vi "AI & AO Synchronization.vi"() -> ()   [LabVIEW 2009, in "MicroDAQ.lvlib"]
uses:
  <instrlib>/MicroDAQ/MicroDAQ.lvlib
  <instrlib>/MicroDAQ/Tools/Analog mode.ctl
  <instrlib>/MicroDAQ/Tools/Analo Range Enum.ctl
  <instrlib>/MicroDAQ/Tools/Analog Channel Enum.ctl
  <instrlib>/MicroDAQ/Tools/Analog input type enum.ctl
  <instrlib>/MicroDAQ/Tools/Analog input Channel enum.ctl
  <instrlib>/MicroDAQ/Tools/External start trigger source.ctl
  <instrlib>/MicroDAQ/Channel/Analog Input/Read NChan NSamp 2D SGL.vi
  <instrlib>/MicroDAQ/Channel/Analog Input/Triggering External start.vi
  <instrlib>/MicroDAQ/Channel/Analog Input/AI Configure Channel.vi
  <instrlib>/MicroDAQ/Channel/Analog Output/Write NChan NSamp 1D Waveform.vi
  <instrlib>/MicroDAQ/Channel/Analog Output/AO Configure Channel.vi
  <instrlib>/MicroDAQ/Channel/Analog Input/Analog Input.lvclass
  <instrlib>/MicroDAQ/Channel/Analog Output/Analog output.lvclass
  <vilib>/measure/NI_MABase.lvlib
panel:
  in  "Sampe Rate":dbl=1000.0
  in  "Samples per channel":dbl=1.0
  out "AI read finish":u32
  out "AI read ready start":u32
  out "AO generation start":u32
  out "AO wait start":u32
  in  "IP address":string="10.10.1.1"
  out "Waveform Graph 2":waveform(dbl)[](graph)=[{"t0"=timestamp(0 s since 1904-01-01), "dt"=0.001, "Y"=[]}]
  out "Waveform Graph":dbl[][](graph)
  # "Device settings"
  # "* All input and output channels settings have been preconfigured as \nconstans to symplify example."
  # "this time should trigger AI start,\nand AI should measure 1000 ms\nand return. So in theory \nAI read finish = AO generation start + 1000ms"
  # "Output signal"
  # "Input signal"
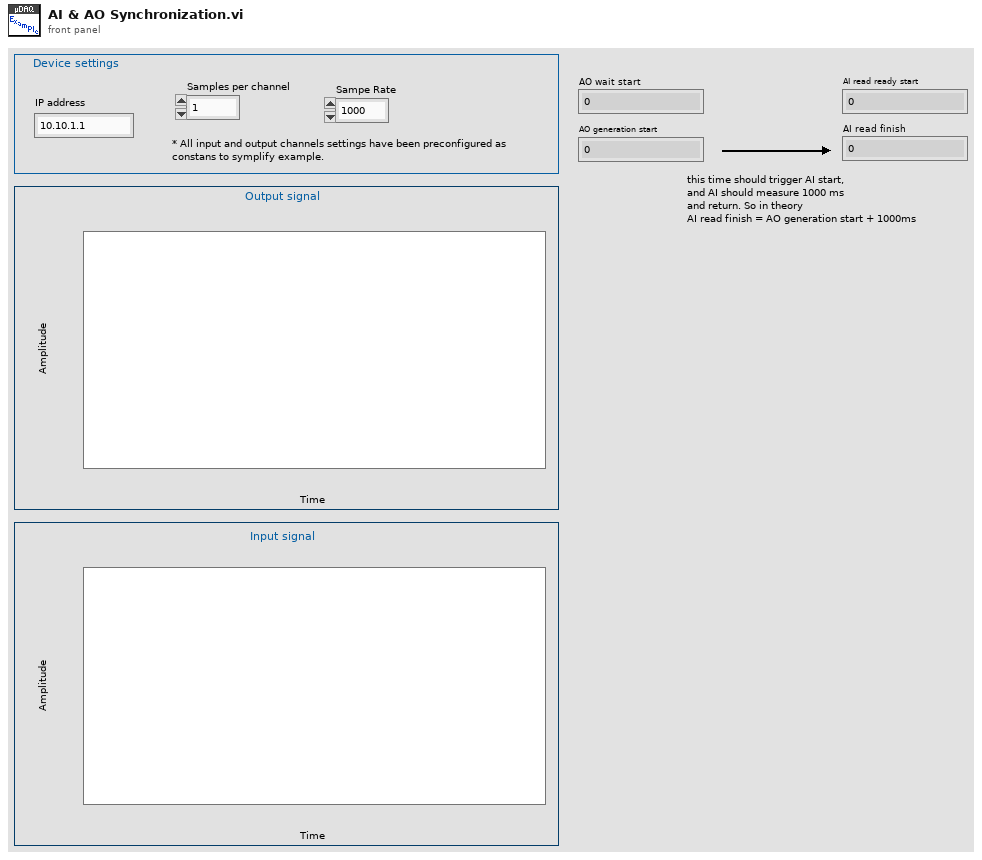
[diagram p1: front panel]
types:
  T1 = typedef "MicroDAQ.lvlib/External start trigger source.ctl" = u16
  T2 = cluster{"Waveform Type":enum16{"Sine Wave", "Triangle Wave", "Square Wave", "Sawtooth Wave"}, "Amplitude":dbl, "Frequency":dbl}[]
  T3 = typedef "MicroDAQ.lvlib/Analog input Channel enum.ctl" = enum16{"None", "AI1", "AI2", "AI3", "AI4", "AI5", "AI6", "AI7", "AI8", "AI9", "AI10", "AI11", "AI12", "AI13", "AI14", "AI15", "AI16"}
  T4 = typedef "MicroDAQ.lvlib/Analo Range Enum.ctl" = enum16{"±10V", "0-10V", "±5V", "0-5V", "±5.12V", "±2.56V", "±2.5V", "±2V", "±1.24V", "±0.64V"}
  T5 = typedef "MicroDAQ.lvlib/Analog input type enum.ctl" = enum16{"Single-ended", "Differential"}
  T6 = typedef "MicroDAQ.lvlib/Analog Channel Enum.ctl" = enum16{"None", "AO1", "AO2", "AO3", "AO4", "AO5", "AO6", "AO7", "AO8", "AO9", "AO10", "AO11", "AO12", "AO13", "AO14", "AO15", "AO16"}
  T7 = typedef "MicroDAQ.lvlib/Analog mode.ctl" = enum16{"Periodic", "Stream"}
  T8 = enum16{"Sine Wave", "Triangle Wave", "Square Wave", "Sawtooth Wave"}
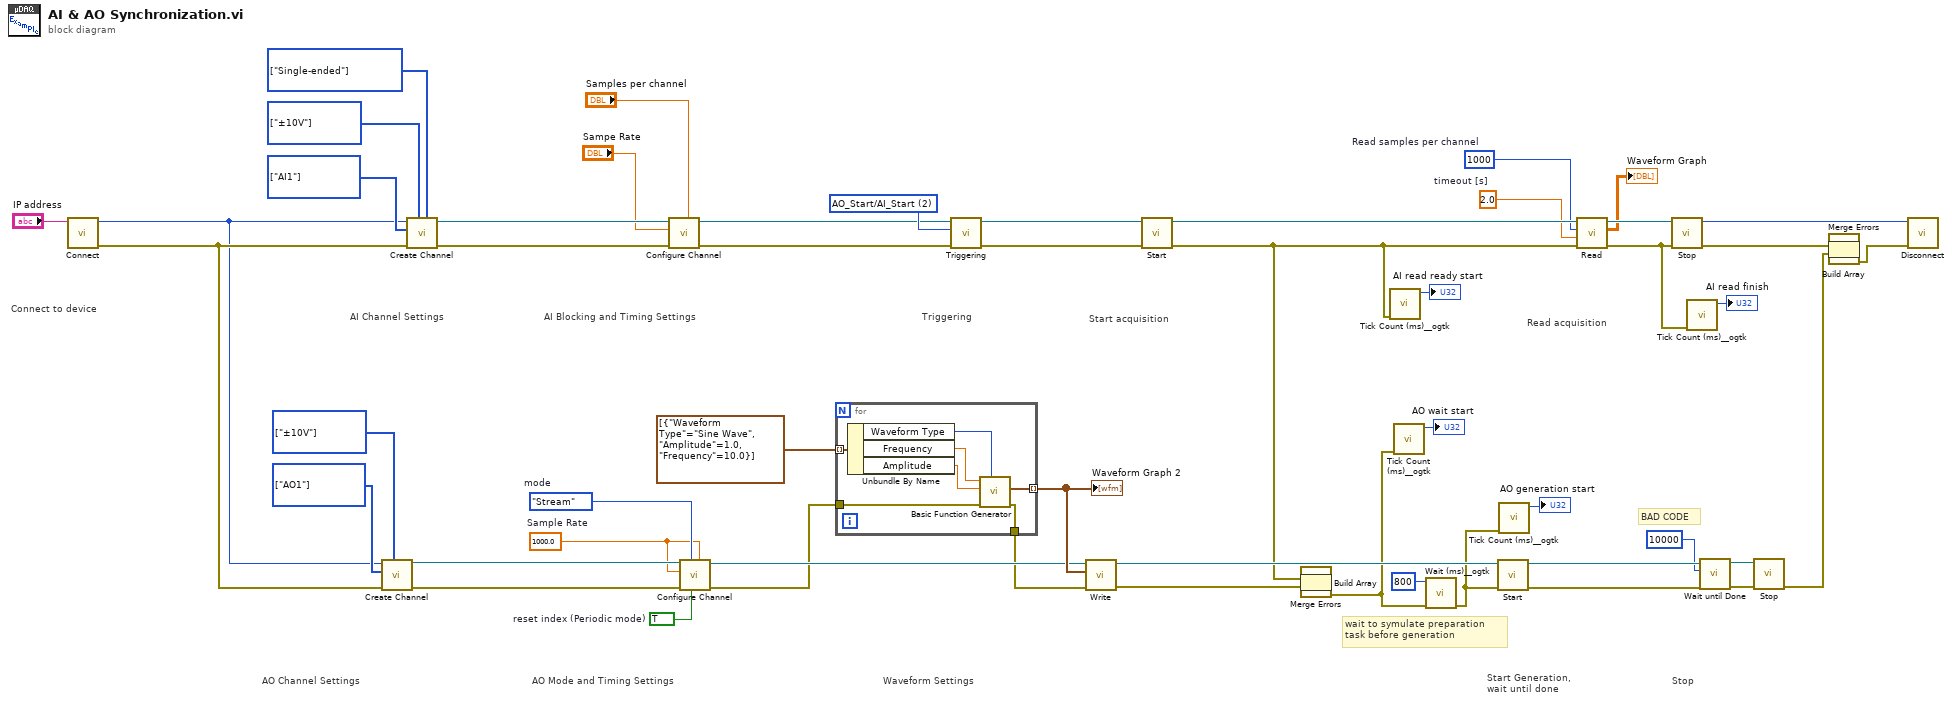
[diagram p0: block diagram]
diagram:
  w20 = T1 2 items=["AO_Start/AI_Start"=2, "DSP_Start"=3] ("source")
  w21 = 2.0  # timeout [s]
  w47 = 1000  # Read samples per channel
  w49 = T3[] [enum."AI1"] items=["None", "AI1", "AI2", "AI3", "AI4", "AI5", "AI6", "AI7", "AI8", "AI9", "AI10", "AI11", "AI12", "AI13", "AI14", "AI15", "AI16"] ("Physical channels")
  w48 = T4[] [enum."±10V"] items=["±10V", "0-10V", "±5V", "0-5V", "±5.12V", "±2.56V", "±2.5V", "±2V", "±1.24V", "±0.64V"] ("Ranges")
  w50 = T5[] [enum."Single-ended"] items=["Single-ended", "Differential"] ("Input terminals configurations")
  w7 = 1000.0  # Sample Rate
  w43 = T6[] [enum."AO1"] items=["None", "AO1", "AO2", "AO3", "AO4", "AO5", "AO6", "AO7", "AO8", "AO9", "AO10", "AO11", "AO12", "AO13", "AO14", "AO15", "AO16"] ("Physical channels 2")
  w42 = T4[] [enum."±10V"] items=["±10V", "0-10V", "±5V", "0-5V", "±5.12V", "±2.56V", "±2.5V", "±2V", "±1.24V", "±0.64V"] ("Ranges 2")
  w38 = TRUE  # reset index (Periodic mode)
  w39 = Analog_mode."Stream"  # mode
  # "wait to symulate preparation \ntask before generation"
  # "BAD CODE"
  # "Start Generation,\nwait until done"
  # "Stop"
  # "Waveform Settings"
  # "AO Mode and Timing Settings"
  # "AO Channel Settings"
  # "Triggering"
  # "Connect to device"
  # "Read acquisition"
  # "Start acquisition"
  # "AI Blocking and Timing Settings"
  # "AI Channel Settings"
  n1 = call <instrlib>:"Connect.vi"("IP address"="IP address") -> ("error out"=w32:errorcluster, "connection ID"=w31:i32)  [unwired: 9 in]
  n2 = call-poly <instrlib>:"Create Channel.vi"("Ranges"=w42, "error in (no error)"=w32, "Phisical channels"=w43, "Connection ID"=w31) -> ("error out"=w40:errorcluster, "Task Out"=w41:refnum<class "Analog output.lvclass">)  [unwired: 6 in]
  n3 = call-poly <instrlib>:"Create Channel.vi"("Input terminals configurations"=w50, "Ranges"=w48, "error in (no error)"=w32, "Phisical channels"=w49, "connection ID"=w31) -> ("error out"=w54:errorcluster, "Task Out"=w4:refnum<class "Analog Input.lvclass">)  [unwired: 5 in]
  n4 = call-poly <instrlib>:"Configure Channel.vi"("Samples per channel"="Samples per channel", "error in (no error)"=w54, "Sampe Rate"="Sampe Rate", "MicroDAQ.lvlib:Analog Input.lvclass"=w4) -> ("error out"=w22:errorcluster, "MicroDAQ.lvlib:Analog Input.lvclass out"=w3:refnum<class "Analog Input.lvclass">)  [unwired: 6 in]
  n5 = call-poly <instrlib>:"Configure Channel.vi"("Samples per channel"=w7, "Reset index (Periodic mode)"=w38, "Mode"=w39, "error in (no error)"=w40, "Sample rate"=w7, "Analog Output in"=w41) -> ("error out"=w29:errorcluster, "Analog Output out"=w30:refnum<class "Analog output.lvclass">)  [unwired: 4 in]
  n6 = for {
    tunnel: [w61] -> w19
    tunnel: T2 [{"Waveform Type"=enum."Sine Wave", "Amplitude"=1.0, "Frequency"=10.0}] ("Waveforms") -> [w60] mode=indexing
    tunnel: [w56] -> w36 mode=indexing
    tunnel: w29 -> [w55]
    n7 = Unbundle By Name(w60) -> ("Waveform Type"=w59:T8, "Frequency"=w58:dbl, "Amplitude"=w57:dbl)
    n8 = call <vilib>:"Basic Function Generator.vi"("signal type"=w59, "error in (no error)"=w55, "amplitude"=w57, "frequency"=w58) -> ("error out"=w61:errorcluster, "signal out"=w56:waveform(dbl))  [unwired: 5 in, 1 out]
  }
  "Waveform Graph 2" <- w36
  n9 = call-poly <instrlib>:"Triggering.vi"("error in (no error)"=w22, "source"=w20, "MicroDAQ.lvlib:Analog Input.lvclass"=w3) -> ("error out"=w44:errorcluster, "MicroDAQ.lvlib:Analog Input.lvclass out"=w45:refnum<class "Analog Input.lvclass">)  [unwired: 7 in]
  n10 = call-poly <instrlib>:"Write.vi"("error in (no error)"=w19, "data"=w36, "Analog Output in"=w30) -> ("error out"=w9:errorcluster, "Analog Output out"=w28:refnum<class "Analog output.lvclass">)  [unwired: 7 in]
  n11 = call-dynamic "Start.vi"("error in (no error)"=w44, "Analog Input in"=w45) -> ("error out"=w8:errorcluster, "Analog Input out"=w53:refnum<class "Analog Input.lvclass">)  [unwired: 8 in]
  n12 = Build Array(w8, w9) -> (w6:errorcluster[])
  n13 = call <vilib>:"Merge Errors.vi"("error array in"=w6) -> ("error out"=w16:errorcluster)  [unwired: 6 in]
  n14 = call <userlib>:"Tick Count (ms)__ogtk.vi"("error in (no error)"=w8) -> ("millisecond timer value"=→"AI read ready start":u32)  [unwired: 9 in, 1 out]
  n15 = call <userlib>:"Tick Count (ms)__ogtk.vi"("error in (no error)"=w16) -> ("millisecond timer value"=→"AO wait start":u32)  [unwired: 9 in, 1 out]
  n16 = call <userlib>:"Wait (ms)__ogtk.vi"("error in (no error)"=w16, "milliseconds to wait"=u32 800) -> ("error out"=w13:errorcluster)  [unwired: 8 in, 1 out]
  n17 = call-dynamic "Start.vi"("error in (no error)"=w13, "Analog Output in"=w28) -> ("error out"=w18:errorcluster, "Analog Output out"=w26:refnum<class "Analog output.lvclass">)  [unwired: 8 in]
  n18 = call <userlib>:"Tick Count (ms)__ogtk.vi"("error in (no error)"=w13) -> ("millisecond timer value"=→"AO generation start":u32)  [unwired: 9 in, 1 out]
  n19 = call-poly <instrlib>:"Read.vi"("error in (no error)"=w8, "timeout [s]"=w21, "number of samples per channel"=w47, "MicroDAQ.lvlib:Analog Input.lvclass"=w53) -> ("error out"=w10:errorcluster, "Values"=→"Waveform Graph":dbl[][], "MicroDAQ.lvlib:Analog Input.lvclass out"=w52:refnum<class "Analog Input.lvclass">)  [unwired: 4 in, 1 out]
  n20 = call-dynamic "Stop.vi"("error in (no error)"=w10, "Analog Input in"=w52) -> ("error out"=w35:errorcluster, "connection ID"=w51:i32)  [unwired: 8 in]
  n21 = call <userlib>:"Tick Count (ms)__ogtk.vi"("error in (no error)"=w10) -> ("millisecond timer value"=→"AI read finish":u32)  [unwired: 9 in, 1 out]
  n22 = call-dynamic "Wait until Done.vi"("error in (no error)"=w18, "timeout [s]"=10000 ("Timeout [ms]"), "Analog output in"=w26) -> ("error out"=w24:errorcluster, "Analog output out"=w25:refnum<class "Analog output.lvclass">)  [unwired: 7 in]
  n23 = call-dynamic "Stop.vi"("error in (no error)"=w24, "Analog Output in"=w25) -> ("error out"=w34:errorcluster)  [unwired: 8 in, 1 out]
  n24 = Build Array(w35, w34) -> (w5:errorcluster[])
  n25 = call <vilib>:"Merge Errors.vi"("error array in"=w5) -> ("error out"=w33:errorcluster)  [unwired: 6 in]
  n26 = call <instrlib>:"Disconnect.vi"("error in (no error)"=w33, "connection ID"=w51) -> ()  [unwired: 9 in, 1 out]
